vi "Temp_dash.vi"() -> ()   [LabVIEW 2023]
doc: "Dashboard to acquring the temprature data and analyse it."
uses:
  LED_details.ctl
panel:
  out "error out":errorcluster
  in  "error in (no error)":errorcluster
  out "State":bool
  in  "Stop_all":bool
  out "Minimum Temp":dbl
  out "Maximum Temp":dbl
  out "Waveform Graph":dbl[](graph)
  out "Chart":dbl(graph)
  out "Low Limit Alert":bool
  out "High Limit Alert":bool
  in  "Start/Stop":bool
  in  "Low Limit":dbl min=0.0 max=100.0
  in  "High Limit":dbl min=0.0 max=100.0
  # "Temperature Monitor"
  # "Acquisition"
  # "Temperature Threshold"
  # "Analysis"
  # "Analysis Data"
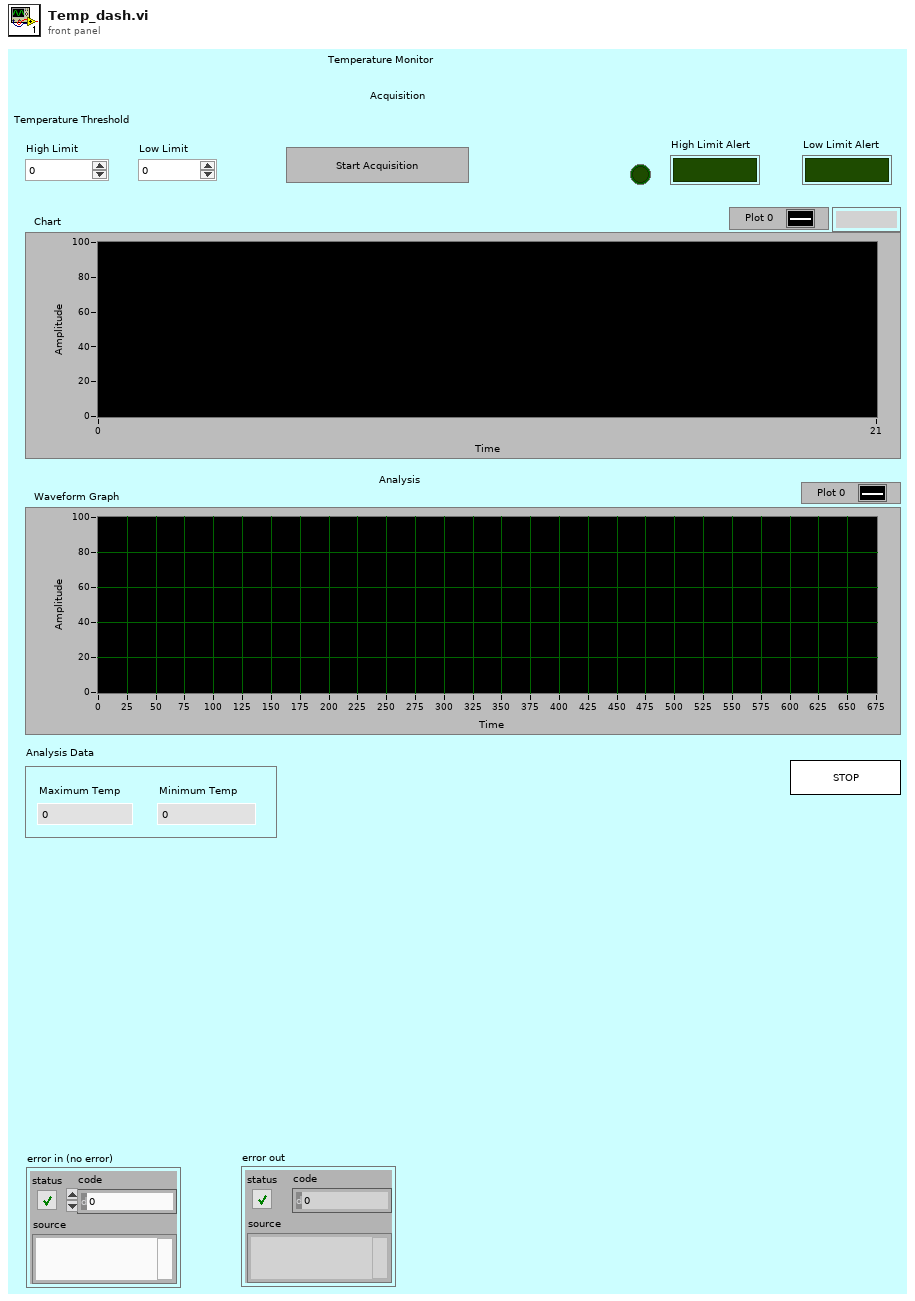
[diagram p1: front panel]
types:
  T1 = typedef "LED_details.ctl" = cluster{"High Limit":dbl, "Low Limit":dbl, "State":bool, "Low Limit Alert":bool, "High Limit Alert":bool}
  T2 = enum8{"Enabled", "Disabled", "Disabled and Grayed Out"}
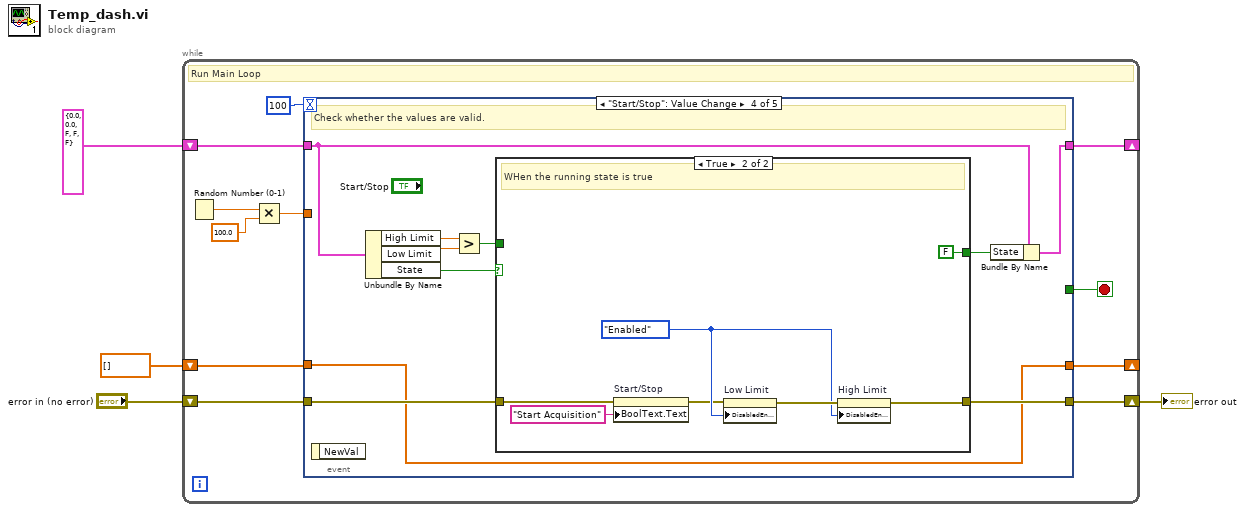
[diagram p0: block diagram]
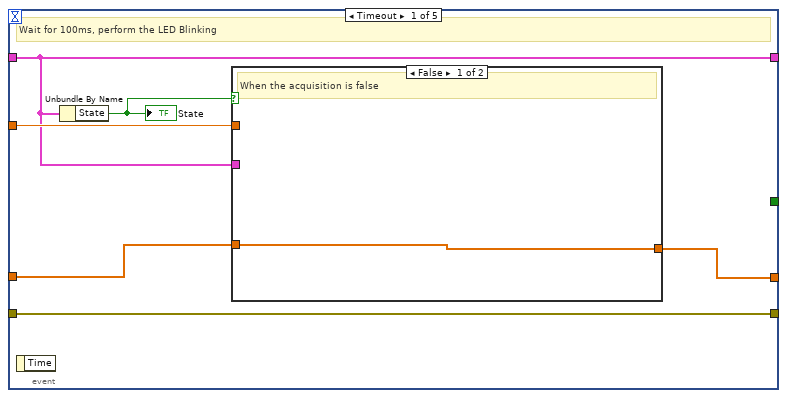
[diagram p2: hidden frame]
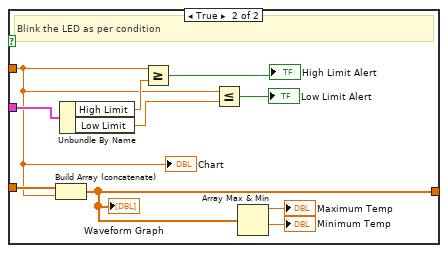
[diagram p3: hidden frame]
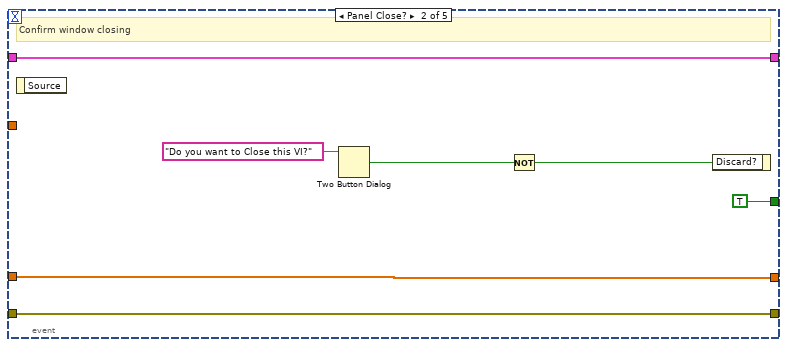
[diagram p4: hidden frame]
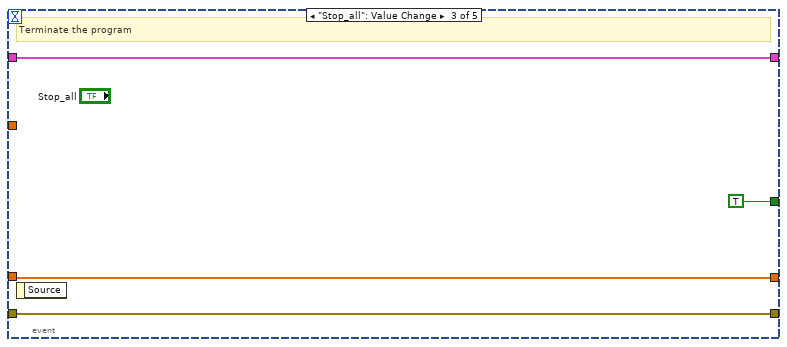
[diagram p5: hidden frame]
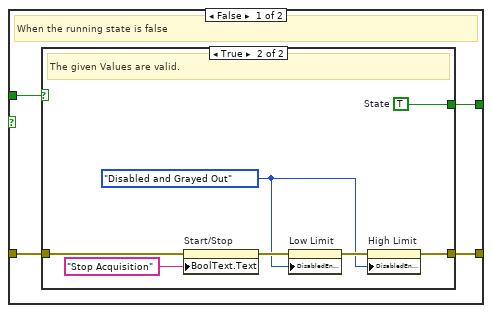
[diagram p6: hidden frame]
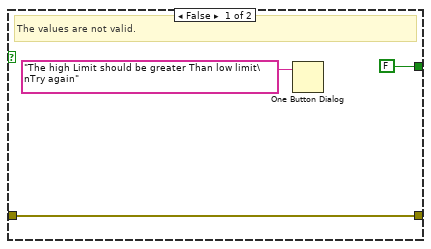
[diagram p7: hidden frame]
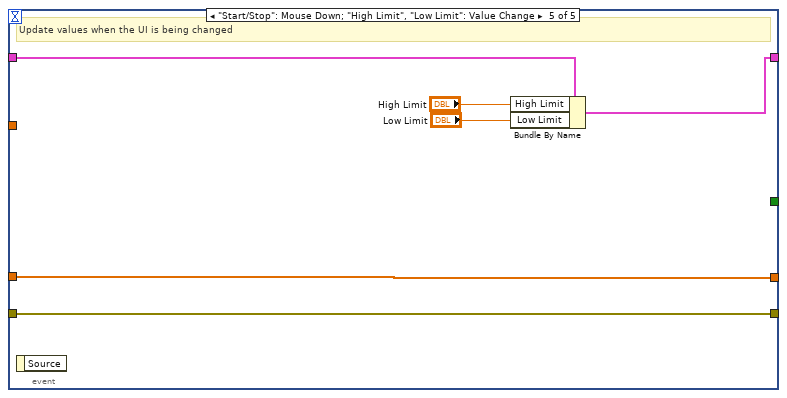
[diagram p8: hidden frame]
diagram:
  n1 = while {
    shift-right: [w7] -> _
    shift-left: dbl[] [] -> [w8]
    shift-right: [w10] -> _
    shift-left: T1 {"High Limit"=0.0, "Low Limit"=0.0, "State"=FALSE, "Low Limit Alert"=FALSE, "High Limit Alert"=FALSE} ("input cluster") -> [w11]
    shift-right: [w5] -> w1
    shift-left: "error in (no error)" -> [w6]
    stop <- w9 stop-if-true
    # "Run Main Loop"
    n2 = Random Number (0-1)() -> (number: 0 to 1=w14:dbl)
    n3 = Multiply(x=w14, y=100.0) -> (x*y=w12:dbl)
    n4 = event shown="[3] \"Start/Stop\": Value Change" {
      selector: _ -> [_ _ _ _ _]
      dyn-events: _ -> [_ _ _ _ _]
      timeout: 100 -> [_ _ _ _ _]
      tunnel: w12 -> [w21 _ _ _ _]
      tunnel: w11 -> [w20 w39 w43 w50 w80]
      tunnel: [w20 w39 w43 w48 w75] -> w10
      tunnel: [_ TRUE TRUE _ _] -> w9
      tunnel: w8 -> [w18 w33 w40 w44 w78]
      tunnel: [w17 w33 w40 w44 w78] -> w7
      tunnel: w6 -> [w16 w34 w41 w46 w79]
      tunnel: [w16 w34 w41 w45 w79] -> w5
      event Timeout {
        # "Wait for 100ms, perform the LED Blinking"
        n5 = event-data() -> ()  [unwired: 1 in, 1 out]
        n6 = Unbundle By Name(w20) -> ("State"=w19:bool)
        "State" <- w19
        n7 = case shown="False" w19 {
          tunnel: w21 -> [_ w24]
          tunnel: w20 -> [_ w30]
          tunnel: w18 -> [w22 w25]
          tunnel: [w22 w23] -> w17
          frame False {
            # "When the acquisition is false"
          }
          frame True {
            # "Blink the LED as per condition"
            n8 = Build Array (concatenate)(w25, w24) -> (w23:dbl[])
            "Waveform Graph" <- w23
            n9 = Unbundle By Name(w30) -> ("High Limit"=w32:dbl, "Low Limit"=w31:dbl)
            n10 = Greater Or Equal?(x=w24, y=w32) -> (x >= y?=→"High Limit Alert":bool)
            n11 = Less Or Equal?(x=w24, y=w31) -> (x <= y?=→"Low Limit Alert":bool)
            n12 = Array Max & Min(array=w23) -> (max value=→"Maximum Temp":dbl, min value=→"Minimum Temp":dbl)  [unwired: 2 out]
            "Chart" <- w24
          }
        }
      }
      event Panel Close? {
        # "Confirm window closing"
        n13 = event-data() -> ()  [unwired: 1 in, 1 out]
        n14 = Two Button Dialog(message="Do you want to Close this VI?") -> (T button?=w37:bool)  [unwired: 2 in]
        n15 = Not(x=w37) -> (.not. x?=w36:bool)
        n16 = event-data("Discard?"=w36) -> ()  [unwired: 1 in, 1 out]
      }
      event "Stop_all": Value Change {
        # "Terminate the program"
        n17 = event-data() -> ()  [unwired: 1 in, 1 out]
      }
      event "Start/Stop": Value Change {
        # "Check whether the values are valid."
        n18 = event-data() -> ()  [unwired: 1 in, 1 out]
        n19 = Unbundle By Name(w50) -> ("High Limit"=w52:dbl, "Low Limit"=w51:dbl, "State"=w47:bool)
        n20 = Greater?(x=w52, y=w51) -> (0:w53:bool)
        n21 = case shown="True" w47 {
          tunnel: w53 -> [w57 _]
          tunnel: [w56 FALSE ("State")] -> w49
          tunnel: w46 -> [w55 w72]
          tunnel: [w54 w68] -> w45
          frame False {
            # "When the running state is false"
            n22 = case shown="True" w57 {
              tunnel: [FALSE w67] -> w56
              tunnel: w55 -> [w58 w66]
              tunnel: [w58 w62] -> w54
              frame False {
                # "The values are not valid."
                n23 = One Button Dialog(message="The high Limit should be greater Than low limit\nTry again") -> ()  [unwired: 1 in, 1 out]
              }
              frame True {
                w61 = T2."Disabled and Grayed Out" ("Disabled")
                w67 = TRUE  # State
                # "The given Values are valid."
                n24 = property on="Start/Stop" class="Bool"(error in=w66, "BoolText.Text"="Stop Acquisition" ("Label.Text")) -> (error out=w64:errorcluster)  [unwired: 1 in, 1 out]
                n25 = property on="Low Limit" class="DigNum (strict)"(error in=w64, "DisabledEnum"=w61) -> (error out=w63:errorcluster)  [unwired: 1 in, 1 out]
                n26 = property on="High Limit" class="DigNum (strict)"(error in=w63, "DisabledEnum"=w61) -> (error out=w62:errorcluster)  [unwired: 1 in, 1 out]
              }
            }
          }
          frame True {
            w70 = T2."Enabled" ("Disabled")
            # "WHen the running state is true"
            n27 = property on="Start/Stop" class="Bool"(error in=w72, "BoolText.Text"="Start Acquisition" ("Label.Text")) -> (error out=w69:errorcluster)  [unwired: 1 in, 1 out]
            n28 = property on="Low Limit" class="DigNum (strict)"(error in=w69, "DisabledEnum"=w70) -> (error out=w71:errorcluster)  [unwired: 1 in, 1 out]
            n29 = property on="High Limit" class="DigNum (strict)"(error in=w71, "DisabledEnum"=w70) -> (error out=w68:errorcluster)  [unwired: 1 in, 1 out]
          }
        }
        n30 = Bundle By Name(cluster=w50, "State"=w49) -> (w48:T1)
      }
      event "Start/Stop": Mouse Down; "High Limit", "Low Limit": Value Change {
        # "Update values when the UI is being changed"
        n31 = event-data() -> ()  [unwired: 1 in, 1 out]
        n32 = Bundle By Name(cluster=w80, "High Limit"="High Limit", "Low Limit"="Low Limit") -> (w75:T1)
      }
    }
  }
  "error out" <- w1
